vi "Create Value - String.vi"(8 "error in (no error)":errorcluster, 10 "String":string) -> (0 "error out":errorcluster, 3 "JSON Tree":variant)   [LabVIEW 2011, in "i3-json.lvlib"]
uses:
  i3-json.lvlib
  JSON Types/JSON Type.ctl
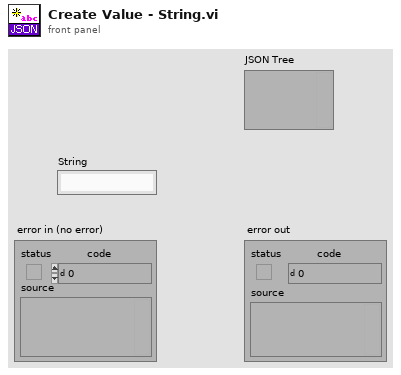
[diagram p1: front panel]
types:
  T1 = typedef "i3-json.lvlib/JSON Type.ctl" = enum8{"JSON Compatible", "JSON Array", "JSON Object", "JSON Null", "Double", "String", "Boolean", "Unknown", "Data JSON string"}
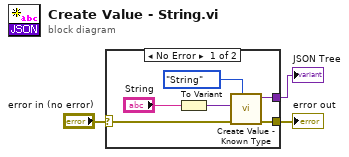
[diagram p0: block diagram]
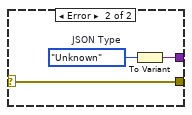
[diagram p2: hidden frame]
diagram:
  n1 = case shown="No Error" "error in (no error)" {
    selector: "error in (no error)" -> [w7 w10]
    tunnel: [w6 w10] -> w2
    tunnel: [w5 w11] -> w1
    frame No Error {
      n2 = To Variant(anything="String") -> (Variant=w8:variant)
      n3 = call "Create Value - Known Type.vi"("JSON Type"=JSON_Type."String", "error in (no error)"=w7, "Value"=w8) -> ("error out"=w6:errorcluster, "JSON Tree"=w5:variant)  [unwired: 7 in]
    }
    frame Error {
      w12 = JSON_Type."Unknown"  # JSON Type
      n4 = To Variant(anything=w12) -> (Variant=w11:variant)
    }
  }
  "JSON Tree" <- w1
  "error out" <- w2
